vi "Cal RHS (VIRef).vi"(8 "error in (no error)":errorcluster, 10 "RHS in":variant, 11 "Domain_Evolut_1D in":refnum<class "NI_Domain_Evolut_1D.lvclass">) -> (0 "error out":errorcluster, 2 "RHS out":variant, 3 "Domain_Evolut_1D out":refnum<class "NI_Domain_Evolut_1D.lvclass">)   [LabVIEW 2020, in "NI_PDE.lvlib" / "NI_Domain_Evolut_1D.lvclass"]
uses:
  <vilib>/gmath/pde.llb/DomainClass/Domain_Evolut_1D/NI_Domain_Evolut_1D.lvclass
  <vilib>/gmath/pde.llb/RHSClass/RHS_2D_VIRef/RHS Data.ctl
  <vilib>/gmath/pde.llb/DomainClass/Domain_Evolut_1D/NI_Domain_Evolut_1D.lvclass/NI_Domain_Evolut_1D.ctl
  <vilib>/Analysis/1siggen.llb/Ramp Pattern by Samples.vi
  <vilib>/gmath/pde.llb/RHSClass/RHS_2D_VIRef/NI_RHS_2D_VIRef.lvclass
  <vilib>/gmath/NI_PDE.lvlib
  <vilib>/Analysis/NI_AALBase.lvlib
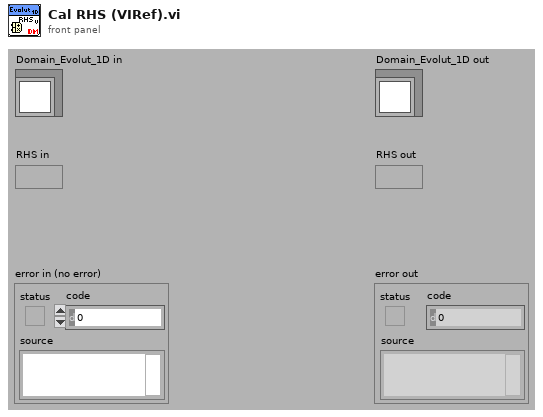
[diagram p1: front panel]
types:
  T1 = typedef "NI_PDE.lvlib/NI_RHS_2D_VIRef.lvclass/RHS Data.ctl" = cluster{"F":refnum<vi>, "data":variant}
  T2 = cluster{"initial t":dbl, "final t":dbl, "# of t-points":i32}
  T3 = cluster{"start x":dbl, "end x":dbl, "# of x-points":i32}
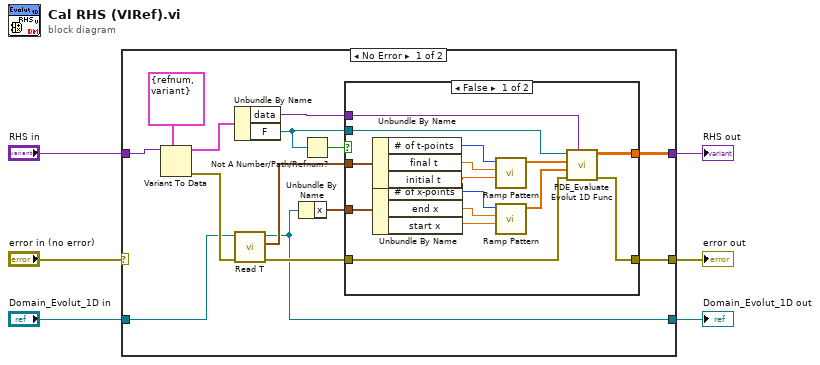
[diagram p0: block diagram]
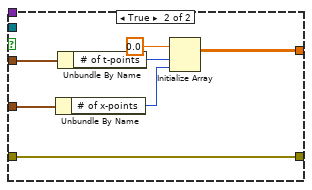
[diagram p2: hidden frame]
diagram:
  n1 = case shown="No Error" "error in (no error)" {
    selector: "error in (no error)" -> [_ w45]
    tunnel: "Domain_Evolut_1D in" -> [w9 w44]
    tunnel: [w7 w44] -> w6
    tunnel: [w11 w45] -> w5
    tunnel: [w10 w43] -> w2
    tunnel: "RHS in" -> [w20 w43]
    frame No Error {
      n2 = Variant To Data(type=T1 {"F"=refnum, "data"=variant} ("RHS data"), Variant=w20) -> (data=w13:T1, error out=w12:errorcluster)  [unwired: 1 in]
      n3 = Unbundle By Name(w13) -> ("data"=w16:variant, "F"=w17:refnum<vi>)
      n4 = call-dynamic "Read T.vi"("error in (no error)"=w12, "Domain_Evolut.lvclass in"=w9) -> ("error out"=w15:errorcluster, "t"=w14:T2, "Domain_Evolut.lvclass out"=w7:refnum<class "NI_Domain_Evolut_1D.lvclass">)  [unwired: 7 out]
      n5 = Unbundle By Name(w7) -> ("x"=w8:T3)
      n6 = Not A Number/Path/Refnum?(number/path/refnum=w17) -> (NaN/Path/Refnum?=w18:bool)
      n7 = case shown="False" w18 {
        tunnel: [w25 w42] -> w10
        tunnel: w14 -> [w35 w41]
        tunnel: w8 -> [w28 w40]
        tunnel: w17 -> [w27 _]
        tunnel: w16 -> [w26 _]
        tunnel: w15 -> [w24 w38]
        tunnel: [w23 w38] -> w11
        frame False {
          n8 = Unbundle By Name(w35) -> ("# of t-points"=w33:i32, "final t"=w32:dbl, "initial t"=w34:dbl)
          n9 = Unbundle By Name(w28) -> ("# of x-points"=w30:i32, "end x"=w31:dbl, "start x"=w29:dbl)
          n10 = call-poly <vilib>:"Ramp Pattern.vi"("start"=w34, "end"=w32, "samples"=w33) -> ("Ramp Pattern"=w22:dbl[])  [unwired: 7 in, 1 out]
          n11 = call-poly <vilib>:"Ramp Pattern.vi"("start"=w29, "end"=w31, "samples"=w30) -> ("Ramp Pattern"=w21:dbl[])  [unwired: 7 in, 1 out]
          n12 = call <vilib>:"PDE_Evaluate Evolut 1D Func.vi"("data"=w26, "error in (no error)"=w24, "X"=w21, "T"=w22, "VIRef"=w27) -> ("error out"=w23:errorcluster, "F(t, x)"=w25:dbl[][])  [unwired: 5 out]
        }
        frame True {
          n13 = Unbundle By Name(w40) -> ("# of x-points"=w36:i32)
          n14 = Unbundle By Name(w41) -> ("# of t-points"=w37:i32)
          n15 = Initialize Array(0.0 ("element"), w37, w36) -> (w42:dbl[][])
        }
      }
    }
    frame Error {
    }
  }
  "Domain_Evolut_1D out" <- w6
  "error out" <- w5
  "RHS out" <- w2
